vi "ImageProcessor.vi"(11 "Microscope in":refnum<class "Microscope.lvclass">) -> (3 "Microscope Out":refnum<class "Microscope.lvclass">)   [LabVIEW 2012]
uses:
  classes/Image.lvclass
  classes/Microscope.lvclass
  typedefs/ImageEvent.ctl
  typedefs/Filenaming.ctl
  variables/GlobalUI.vi
  methods/ImageUpdateImage-2D.vi
  methods/ImageReadImage-2D.vi
  methods/ImageSaveImage-2D.vi
panel:
  in  "Image in":refnum<class "Image.lvclass">
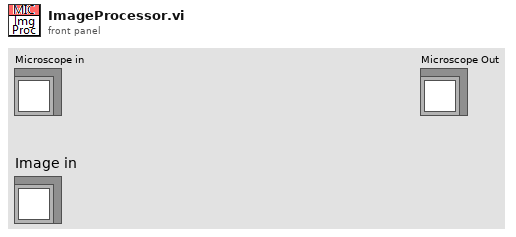
[diagram p1: front panel]
types:
  T1 = typedef "ImageEvent.ctl" = enum16{"i.Wait", "i.Acquire", "i.InitImageData", "i.ReinitImageData", "i.ReinitImageParams", "i.PreAcquire", "i.PostAcquire", "i.ClearData"}
  T2 = typedef "Filenaming.ctl" = enum16{"Image", "Just Description"}
  T3 = typedef "Stage Parameters.ctl" = cluster{"Scan Mode":T4, "Start position mm":dbl, "End position mm":dbl, "Velocity um/sec (continuous)":dbl, "Step size microns (discrete)":dbl, "Frames to grab (grab)":i32}
  T4 = typedef "ScanMode.ctl" = enum16{"None", "Continuous", "Point Scan (CH3 cursor)", "Point Scan Move (CH3 cursor)", "Grab", "Grab Move Stage", "Grab Move Z-stage", "Cont. Move Z-stage", "Spec Move Stage", "Spec Move Cont", "Surf Calib"}
  T5 = typedef "HWsettings.ctl" = cluster{"Galvo Channels":tag, "Detector Channels":tag, "Galvo Trigger":tag, "Shutter Lines":tag[], "Max Acquisition Rate":dbl, "Recommended Acquisition Rate":dbl, "Galvo Write Rate":dbl, "Max Timebase Frequency (Hz)":dbl, "MCC Shutter Lines":refnum<k21>[], "Detector Task":refnum<k21>, "Shutter Tasks":refnum<k21>[], "Galvo Task":refnum<k21>, "Digital Image Multiplier":dbl[]}
  T6 = typedef "Scan Parameters.ctl" = cluster{"x pixels":i32, "x voltage min":dbl, "x voltage max":dbl, "y voltage min":dbl, "y voltage max":dbl, "fill frac":dbl, "Zoom":dbl, "BiDi":bool, "scan rate (ms/line)":dbl}
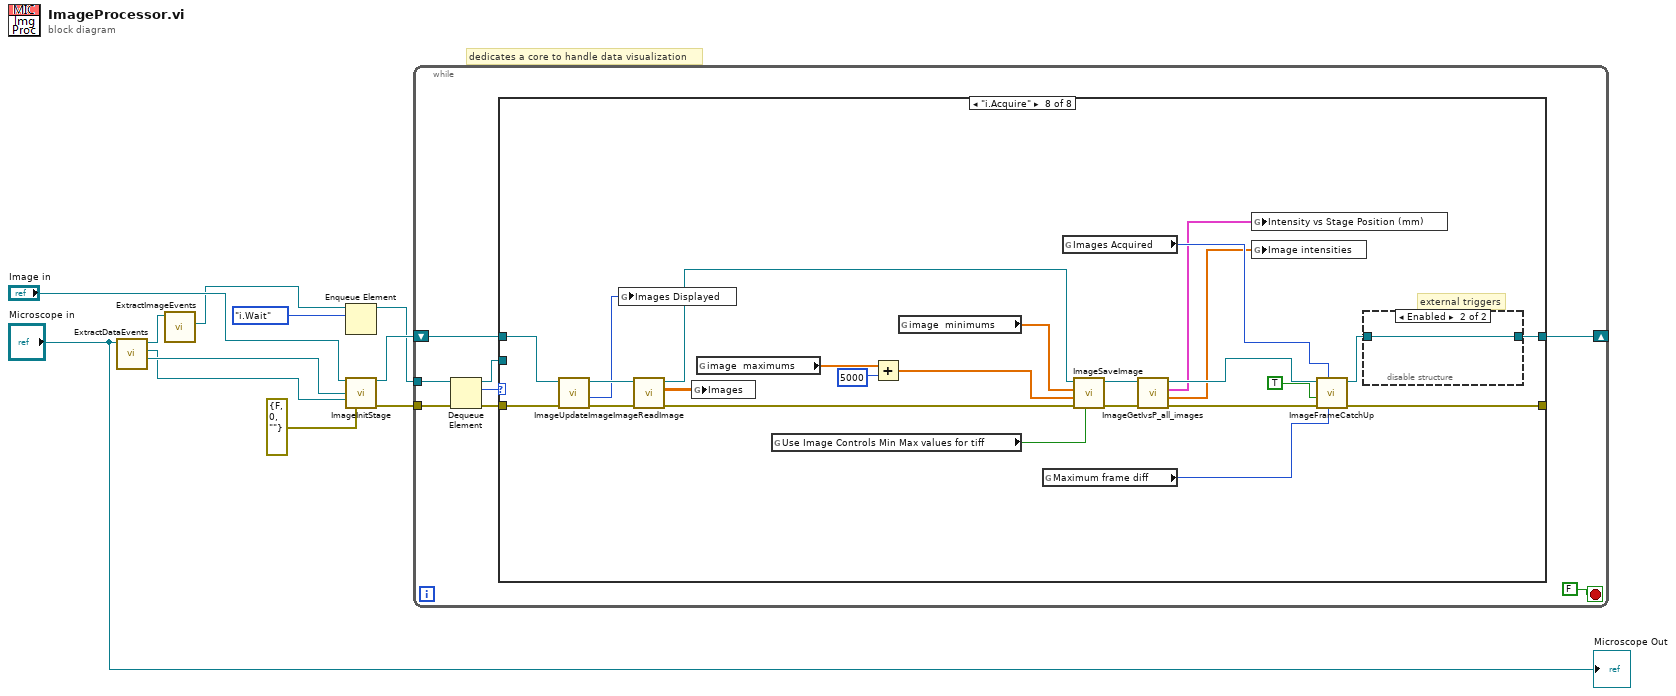
[diagram p0: block diagram]
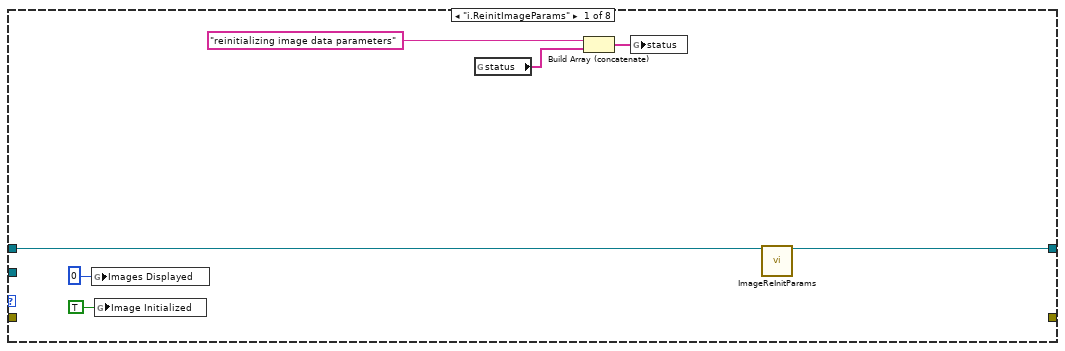
[diagram p2: hidden frame]
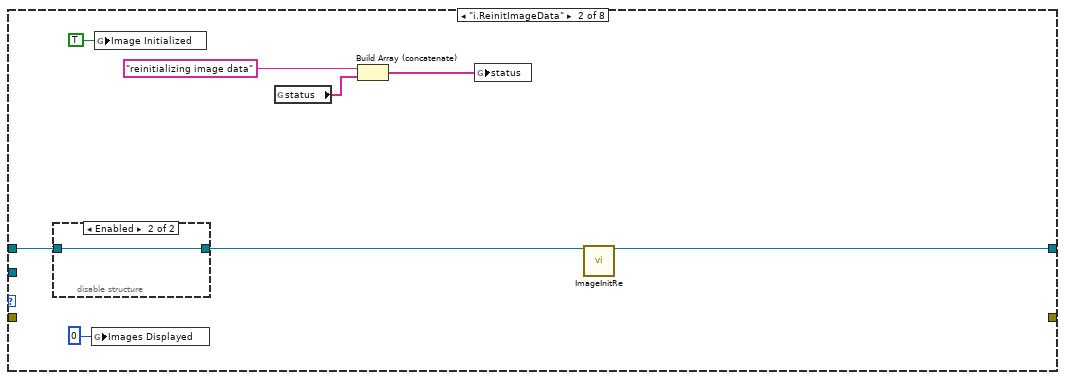
[diagram p3: hidden frame]
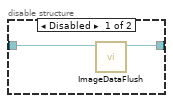
[diagram p4: hidden frame]
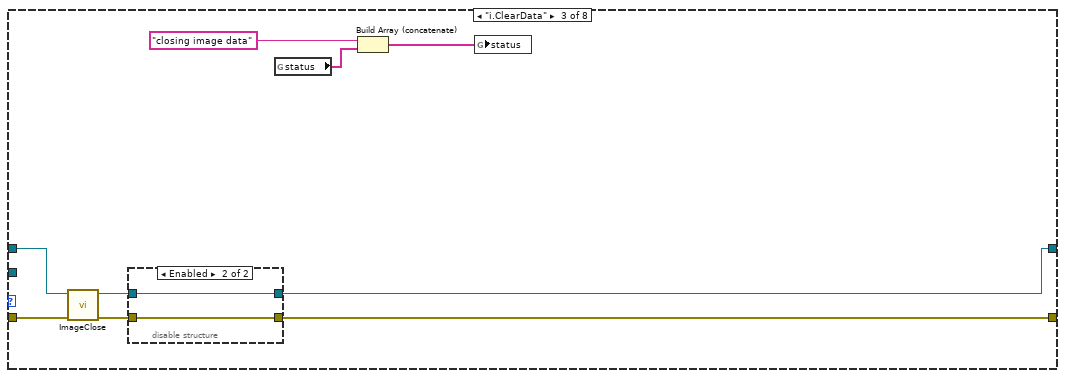
[diagram p5: hidden frame]
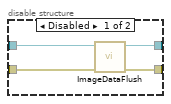
[diagram p6: hidden frame]
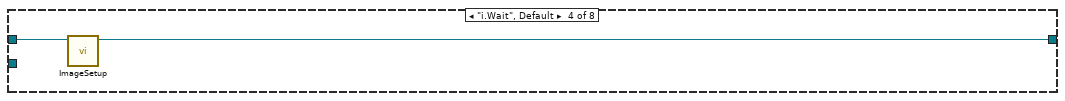
[diagram p7: hidden frame]
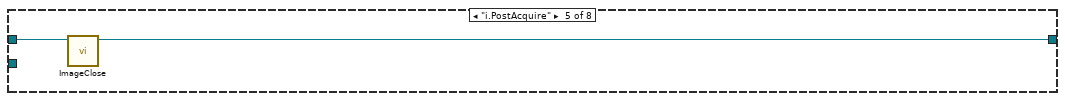
[diagram p8: hidden frame]
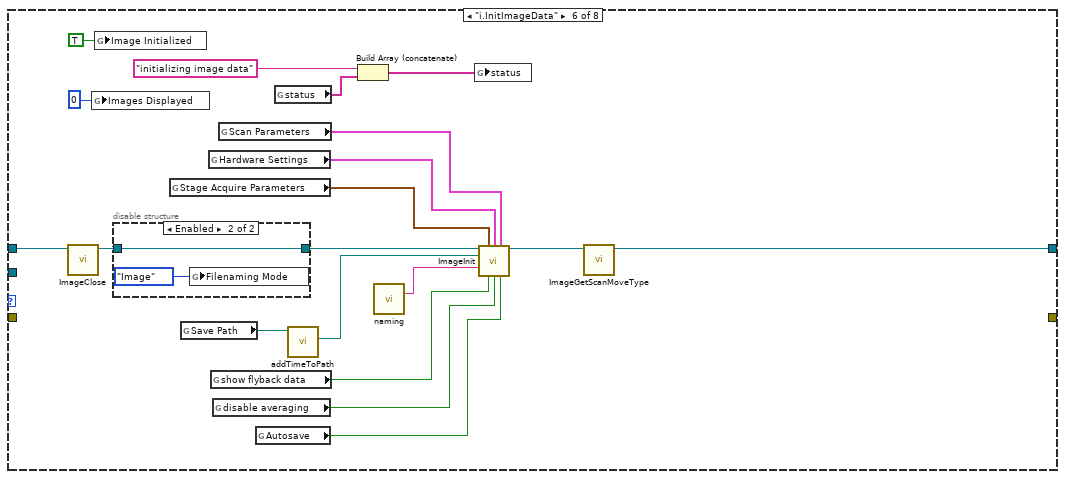
[diagram p9: hidden frame]
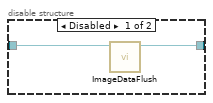
[diagram p10: hidden frame]
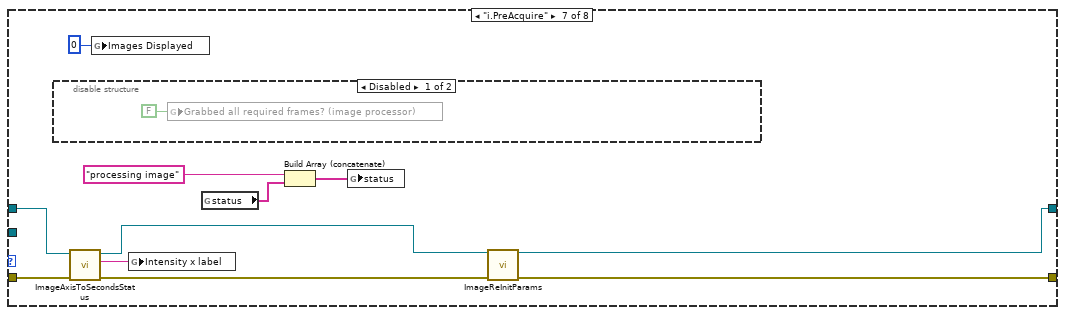
[diagram p11: hidden frame]
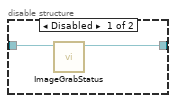
[diagram p13: hidden frame]
diagram:
  # "dedicates a core to handle data visualization"
  n1 = call "ExtractDataEvents.vi"("Microscope in"="Microscope in") -> ("Raw Data"=w7:refnum<queue>, "X Data"=w6:refnum<queue>, "Microscope out"=w9:refnum<class "Microscope.lvclass">)  [unwired: 7 in, 1 out]
  n2 = call "ExtractImageEvents.vi"("Microscope in"=w9) -> ("Image events"=w3:refnum<queue>)  [unwired: 8 in, 2 out]
  n3 = Enqueue Element(queue=w3, element=ImageEvent."i.Wait") -> (queue out=w1:refnum<queue>)  [unwired: 2 in, 2 out]
  n4 = call "ImageInitStage.vi"("Image in"="Image in", "data queue"=w7, "Stage Data queue"=w6, "error in (no error)"=errorcluster {"status"=FALSE, "code"=0, "source"=""}) -> ("Image out"=w10:refnum<class "Image.lvclass">, "error out"=w5:errorcluster)  [unwired: 10 in]
  n5 = while {
    shift-right: [w17] -> _
    shift-left: w10 -> [w16]
    tunnel: w1 -> [w15]
    tunnel: w5 -> [w12]
    stop <- FALSE stop-if-true
    n6 = Dequeue Element(queue=w15, error in (no error)=w12) -> (queue out=w14:refnum<queue>, element=w18:T1, error out=w13:errorcluster)  [unwired: 1 in, 1 out]
    n7 = case shown="\"i.Acquire\"" w18 {
      tunnel: w16 -> [w26 w29 w46 w54 w56 w61 w88 w115]
      tunnel: [w25 w30 w44 w53 w55 w60 w89 w116] -> w17
      tunnel: w14 -> [_ _ _ _ _ _ _ _]
      tunnel: w13 -> [_ _ w39 _ _ _ w82 w95]
      tunnel: [_ _ w38 _ _ _ w80 w96] -> _
      frame "i.ReinitImageParams" {
        n8 = global write "GlobalUI.vi" "Images Displayed"(0 ("Frames grabbed")) -> ()
        n9 = global write "GlobalUI.vi" "Image Initialized"(TRUE ("Image Initialized")) -> ()
        n10 = global read "GlobalUI.vi" "status"() -> (w23:string[])
        n11 = Build Array (concatenate)("reinitializing image data parameters" ("status"), w23) -> (w22:string[])
        n12 = global write "GlobalUI.vi" "status"(w22) -> ()
        n13 = call "ImageReInitParams.vi"("Image in"=w26) -> ("Image out"=w25:refnum<class "Image.lvclass">)  [unwired: 13 in, 1 out]
      }
      frame "i.ReinitImageData" {
        n14 = disable-structure shown="Enabled" {
          disable-tunnel: w29 -> [w36 w37]
          disable-tunnel: [w35 w37] -> w28
          frame Disabled {
            n15 = call "ImageDataFlush.vi"("Image in"=w36) -> ("Image out"=w35:refnum<class "Image.lvclass">)  [unwired: 9 in, 1 out]
          }
          frame Enabled {
          }
        }
        n16 = global write "GlobalUI.vi" "Images Displayed"(0 ("Images Acquired")) -> ()
        n17 = global write "GlobalUI.vi" "Image Initialized"(TRUE ("Image Initialized")) -> ()
        n18 = global read "GlobalUI.vi" "status"() -> (w33:string[])
        n19 = Build Array (concatenate)("reinitializing image data" ("status"), w33) -> (w32:string[])
        n20 = global write "GlobalUI.vi" "status"(w32) -> ()
        n21 = call "ImageInitRe.vi"("Image in"=w28) -> ("Image out"=w30:refnum<class "Image.lvclass">)  [unwired: 13 in, 1 out]
      }
      frame "i.ClearData" {
        n22 = call "ImageClose.vi"("error in (no error)"=w39, "Image in"=w46) -> ("error out"=w40:errorcluster, "Image out"=w45:refnum<class "Image.lvclass">)  [unwired: 8 in]
        n23 = disable-structure shown="Enabled" {
          disable-tunnel: w45 -> [w50 w52]
          disable-tunnel: [w49 w52] -> w44
          disable-tunnel: w40 -> [w48 w51]
          disable-tunnel: [w47 w51] -> w38
          frame Disabled {
            n24 = call "ImageDataFlush.vi"("error in (no error)"=w48, "Image in"=w50) -> ("error out"=w47:errorcluster, "Image out"=w49:refnum<class "Image.lvclass">)  [unwired: 8 in]
          }
          frame Enabled {
          }
        }
        n25 = global read "GlobalUI.vi" "status"() -> (w43:string[])
        n26 = Build Array (concatenate)("closing image data" ("status"), w43) -> (w42:string[])
        n27 = global write "GlobalUI.vi" "status"(w42) -> ()
      }
      frame "i.Wait", Default {
        n28 = call "ImageSetup.vi"("Image in"=w54) -> ("Image out"=w53:refnum<class "Image.lvclass">)  [unwired: 9 in, 1 out]
      }
      frame "i.PostAcquire" {
        n29 = call "ImageClose.vi"("Image in"=w56) -> ("Image out"=w55:refnum<class "Image.lvclass">)  [unwired: 9 in, 1 out]
      }
      frame "i.InitImageData" {
        n30 = call "ImageClose.vi"("Image in"=w61) -> ("Image out"=w62:refnum<class "Image.lvclass">)  [unwired: 9 in, 1 out]
        n31 = global write "GlobalUI.vi" "Images Displayed"(0 ("Frames grabbed")) -> ()
        n32 = global write "GlobalUI.vi" "Image Initialized"(TRUE ("Image Initialized")) -> ()
        n33 = disable-structure shown="Enabled" {
          disable-tunnel: [w77 w79] -> w63
          disable-tunnel: w62 -> [w76 w79]
          frame Disabled {
            n34 = call "ImageDataFlush.vi"("Image in"=w76) -> ("Image out"=w77:refnum<class "Image.lvclass">)  [unwired: 9 in, 1 out]
          }
          frame Enabled {
            n35 = global write "GlobalUI.vi" "Filenaming Mode"(Filenaming."Image" ("Filenaming Mode")) -> ()
          }
        }
        n36 = global read "GlobalUI.vi" "Stage Acquire Parameters"() -> (w64:T3)
        n37 = global read "GlobalUI.vi" "Save Path"() -> (w59:path)
        n38 = global read "GlobalUI.vi" "Hardware Settings"() -> (w73:T5)
        n39 = global read "GlobalUI.vi" "show flyback data"() -> (w70:bool)
        n40 = global read "GlobalUI.vi" "disable averaging"() -> (w68:bool)
        n41 = global read "GlobalUI.vi" "Scan Parameters"() -> (w72:T6)
        n42 = global read "GlobalUI.vi" "Autosave"() -> (w69:bool)
        n43 = global read "GlobalUI.vi" "status"() -> (w67:string[])
        n44 = call "addTimeToPath.vi"("Path"=w59) -> ("Time Path (Path)"=w58:path)  [unwired: 9 in, 1 out]
        n45 = Build Array (concatenate)("initializing image data" ("status"), w67) -> (w66:string[])
        n46 = call "naming.vi"() -> ("filename"=w75:string)  [unwired: 15 in]
        n47 = global write "GlobalUI.vi" "status"(w66) -> ()
        n48 = call "ImageInit.vi"("Image in"=w63, "Stage Acquire Parameters"=w64, "Hardware Settings"=w73, "Scan Parameters"=w72, "Save Path"=w58, "Filename"=w75, "show flyback data"=w70, "disable averaging"=w68, "Autosave"=w69) -> ("Image out"=w65:refnum<class "Image.lvclass">)  [unwired: 5 in, 1 out]
        n49 = call "ImageGetScanMoveType.vi"("Image in"=w65) -> ("Image out"=w60:refnum<class "Image.lvclass">)  [unwired: 9 in, 1 out]
      }
      frame "i.PreAcquire" {
        n50 = disable-structure shown="Disabled" {
          frame Disabled {
            n51 = global write "GlobalUI.vi" "Grabbed all required frames? (image processor)"(FALSE ("Grabbed all required frames? (view)")) -> ()
          }
          frame Enabled {
          }
        }
        n52 = call "ImageAxisToSecondsStatus.vi"("error in (no error)"=w82, "Image in"=w88) -> ("error out"=w81:errorcluster, "Intensity x label"=w83:string, "Image out"=w90:refnum<class "Image.lvclass">)  [unwired: 7 in]
        n53 = global write "GlobalUI.vi" "Images Displayed"(0 ("Frames grabbed")) -> ()
        n54 = global write "GlobalUI.vi" "Intensity x label"(w83) -> ()
        n55 = global read "GlobalUI.vi" "status"() -> (w86:string[])
        n56 = Build Array (concatenate)("processing image" ("status"), w86) -> (w85:string[])
        n57 = global write "GlobalUI.vi" "status"(w85) -> ()
        n58 = call "ImageReInitParams.vi"("Image in"=w90, "error in (no error)"=w81) -> ("Image out"=w89:refnum<class "Image.lvclass">, "error out"=w80:errorcluster)  [unwired: 12 in]
      }
      frame "i.Acquire" {
        # "external triggers"
        n59 = call-poly "ImageUpdateImage.vi"("error in (no error)"=w95, "Image in"=w115) -> ("error out"=w100:errorcluster, "Images Displayed"=w106:i32, "Image out"=w114:refnum<class "Image.lvclass">)  [unwired: 7 in]
        n60 = global write "GlobalUI.vi" "Images Displayed"(w106) -> ()
        n61 = call-poly "ImageReadImage.vi"("error in (no error)"=w100, "Image in"=w114) -> ("error out"=w99:errorcluster, "Images"=w103:dbl[][][], "Image out"=w113:refnum<class "Image.lvclass">)  [unwired: 7 in]
        n62 = global write "GlobalUI.vi" "Images"(w103) -> ()
        n63 = global read "GlobalUI.vi" "image  maximums"() -> (w94:dbl[])
        n64 = global read "GlobalUI.vi" "Use Image Controls Min Max values for tiff"() -> (w105:bool)
        n65 = Add(x=w94, y=5000) -> (x+y=w92:dbl[])
        n66 = global read "GlobalUI.vi" "image  minimums"() -> (w108:dbl[])
        n67 = global read "GlobalUI.vi" "Maximum frame diff"() -> (w104:i32)
        n68 = global read "GlobalUI.vi" "Images Acquired"() -> (w107:i32)
        n69 = call-poly "ImageSaveImage.vi"("Modify Min Max"=w105, "error in (no error)"=w99, "Maxs"=w92, "Mins"=w108, "Image in"=w113) -> ("error out"=w98:errorcluster, "Image out"=w112:refnum<class "Image.lvclass">)  [unwired: 5 in]
        n70 = call "ImageGetIvsP_all_images.vi"("error in (no error)"=w98, "Image in"=w112) -> ("error out"=w97:errorcluster, "Added Image Intensity (I_new)"=w102:dbl[], "Intensity vs Stage Position (mm)"=w101:cluster{dbl[], dbl[]}[], "Image out"=w111:refnum<class "Image.lvclass">)  [unwired: 6 in]
        n71 = global write "GlobalUI.vi" "Intensity vs Stage Position (mm)"(w101) -> ()
        n72 = global write "GlobalUI.vi" "Image intensities"(w102) -> ()
        n73 = call "ImageFrameCatchUp.vi"("Frame Diff Limit"=w104, "Images Acquired"=w107, "error in (no error)"=w97, "Enable"=TRUE, "Image in"=w111) -> ("error out"=w96:errorcluster, "Image out"=w110:refnum<class "Image.lvclass">)  [unwired: 4 in, 1 out]
        n74 = disable-structure shown="Enabled" {
          disable-tunnel: [w118 w119] -> w116
          disable-tunnel: w110 -> [w117 w119]
          frame Disabled {
            n75 = call "ImageGrabStatus.vi"("Image in"=w117) -> ("Image out"=w118:refnum<class "Image.lvclass">)  [unwired: 8 in, 2 out]
          }
          frame Enabled {
          }
        }
      }
    }
  }
  "Microscope Out" <- "Microscope in"
